vi "Read FPSZ.vi"(3 "FP":refnum<class "DecFrame_FP.lvclass">) -> (1 "Size Out":refnum<class "GObject_FPSZ.lvclass">)   [LabVIEW 2020, in "DecFrame_FP.lvclass"]
uses:
  DecFrame_FP/DecFrame_FP.lvclass
  GObject_FPSZ/GObject_FPSZ.lvclass
  DecFrame_FP/DecFrame_FP.lvclass/DecFrame_FP.ctl
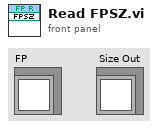
[diagram p1: front panel]
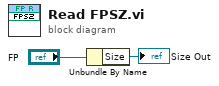
[diagram p0: block diagram]
diagram:
  n1 = Unbundle By Name("FP") -> ("Size"=→"Size Out":refnum<class "GObject_FPSZ.lvclass">)
